vi "Sensor Data.vi"   [LabVIEW 2012, in "Lake Shore 335.lvlib"]
uses:
  <instrlib>/lake shore 335/Temperature control panel Folder/C/Program Files/National Instruments/LabVIEW 2013/instr.lib/lake shore 335/Lake Shore 335.lvlib
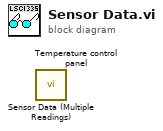
[diagram p0: block diagram]
diagram:
  n1 = call <instrlib>:"Sensor Data (Multiple Readings).vi"() -> ()  [unwired: 9 in, 3 out]
  n2 = call <instrlib>:"Temperature control panel.vi"() -> ()  [unwired: 9 in, 3 out]
